vi "CreateValidFilePath (SubVI).vi"(9 "file name (no extension)":string, 10 "folder  name":string) -> (3 "path":path)   [LabVIEW 2025]
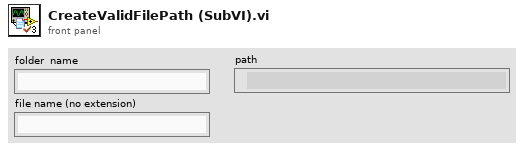
[diagram p1: front panel]
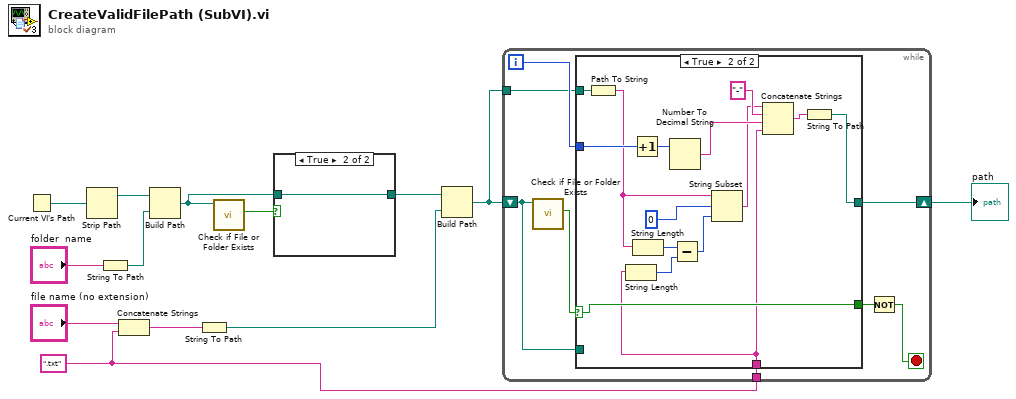
[diagram p0: block diagram]
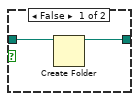
[diagram p3: hidden frame]
diagram:
  w2 = ".txt"
  n1 = Current VI's Path() -> (path=w8:path)
  n2 = Strip Path(path=w8) -> (stripped path=w9:path)  [unwired: 1 out]
  n3 = String To Path(string="folder  name") -> (path=w6:path)
  n4 = Concatenate Strings("file name (no extension)", w2) -> (w1:string)
  n5 = Build Path(base path=w9, name or relative path=w6) -> (appended path=w11:path)
  n6 = String To Path(string=w1) -> (path=w4:path)
  n7 = call <vilib>:"Check if File or Folder Exists.vi"("path"=w11) -> ("file or folder exists?"=w10:bool)  [unwired: 8 in, 2 out]
  n8 = case shown="True" w10 {
    tunnel: w11 -> [w15 w16]
    tunnel: [w14 w16] -> w12
    frame False {
      n9 = Create Folder(path (use dialog)=w15) -> (created path=w14:path)  [unwired: 2 in, 2 out]
    }
    frame True {
    }
  }
  n10 = Build Path(base path=w12, name or relative path=w4) -> (appended path=w13:path)
  n11 = while {
    shift-right: [w23] -> w7
    shift-left: w13 -> [w18]
    tunnel: w13 -> [w22]
    tunnel: w2 -> [w17]
    i -> [w24]
    stop <- w19 stop-if-true
    n12 = call <vilib>:"Check if File or Folder Exists.vi"("path"=w18) -> ("file or folder exists?"=w21:bool)  [unwired: 8 in, 2 out]
    n13 = case shown="True" w21 {
      selector: w21 -> [w26 w28]
      tunnel: w24 -> [_ w41]
      tunnel: [w25 w29] -> w23
      tunnel: w22 -> [_ w30]
      tunnel: [w26 w28] -> w20
      tunnel: w18 -> [w25 _]
      tunnel: w17 -> [_ w27]
      frame False {
      }
      frame True {
        n14 = Path To String(path=w30) -> (string=w36:string)
        n15 = String Length(string=w27) -> (length=w31:i32)
        n16 = Increment(x=w41) -> (x+1=w39:i32)
        n17 = String Length(string=w36) -> (length=w35:i32)
        n18 = Number To Decimal String(number=w39) -> (decimal integer string=w38:string)  [unwired: 1 in]
        n19 = Subtract(x=w35, y=w31) -> (x-y=w33:i32)
        n20 = String Subset(string=w36, offset (0)=0, length (rest)=w33) -> (substring=w32:string)
        n21 = Concatenate Strings(w32, "-", w38, w27) -> (w37:string)
        n22 = String To Path(string=w37) -> (path=w29:path)
      }
    }
    n23 = Not(x=w20) -> (.not. x?=w19:bool)
  }
  "path" <- w7
